vi "Flatten 2D to 1D.vi"(11 "Image Pixels (U32) in":u32[][](array[numeric])) -> (3 "Image Pixels (U32) out":u32[](array[numeric]))   [LabVIEW 2013]
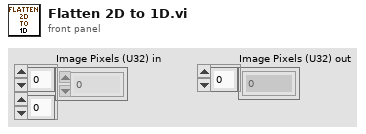
[diagram p1: front panel]
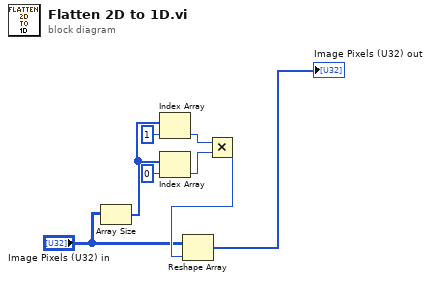
[diagram p0: block diagram]
diagram:
  n1 = Array Size(array="Image Pixels (U32) in") -> (size(s)=w5:i32[])
  n2 = Index Array(array=w5, index=1) -> (element=w7:i32)
  n3 = Index Array(array=w5, index=0) -> (element=w6:i32)
  n4 = Multiply(x=w7, y=w6) -> (x*y=w8:i32)
  n5 = Reshape Array("Image Pixels (U32) in", w8) -> (→"Image Pixels (U32) out":u32[])
